vi "Get Date Time String.vi"(11 "Time (Current time)":timestamp) -> (3 "Time String":string)   [LabVIEW 2019, in "ProjectBuilder.lvlib"]
doc: "Return date/time as a string with the following format: %<%Y-%m-%d %H.%M.%S>T"
uses:
  ProjectBuilder.lvlib
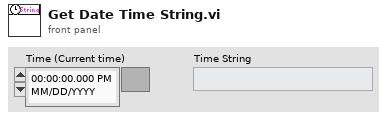
[diagram p1: front panel]
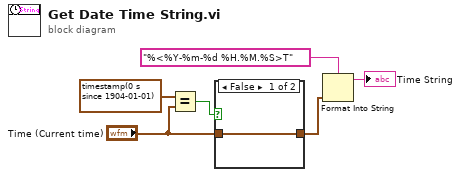
[diagram p0: block diagram]
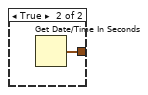
[diagram p2: hidden frame]
diagram:
  n1 = Equal?(x=timestamp(0 s since 1904-01-01) ("current time"), y="Time (Current time)") -> (x = y?=w2:bool)
  n2 = case shown="False" w2 {
    tunnel: [w7 w8] -> w4
    tunnel: "Time (Current time)" -> [w7 _]
    frame False {
    }
    frame True {
      n3 = Get Date/Time In Seconds() -> (seconds since 1Jan1904=w8:timestamp)
    }
  }
  n4 = Format Into String(format string="%<%Y-%m-%d %H.%M.%S>T" ("initial string"), w4) -> (resulting string=→"Time String":string)  [unwired: 2 in, 1 out]
